vi "Lake Shore Cryotronics 218 Alarm Configuration.vi"() -> ()   [LabVIEW 2017]
doc: "This example VI demonstrates the use of the Alarm VIs to configure the Alarm function and monitor the Alarm Status for the selected input. A typical use of this example would be to configure the Alarm functions the first time this is run and then monitor the Alarm status by running this VI in a loop."
uses:
  Lake Shore Cryotronics 218.lvlib
panel:
  out "VISA resource name out":refnum<visa-resource-name>
  out "error out":errorcluster
  in  "error in (no error)":errorcluster
  in  "VISA resource name":refnum<visa-resource-name>
  out "Beeper Status (F)":bool
  out "Alarm Low Status (F)":bool
  out "Alarm High Status (F)":bool
  in  "Beeper (F: Beeper Disabled)":bool
  in  "Latching (F: Alarm Latch OFF)":bool
  in  "Alarm (F: Alarm Disabled)":bool
  in  "Deadband (0.0000)":dbl min=0.0 max=9999.9 step=0.0001 format="%.4f"
  in  "Low Value (0.0000)":dbl min=-9999.9 max=9999.9 step=0.0001 format="%.4f"
  in  "High Value (0.0000)":dbl min=-9999.9 max=9999.9 step=0.0001 format="%.4f"
  in  "Alarm Source (0:Kelvin)":u16(ring) items=["Kelvin", "Celsius", "Sensor Units", "Linear Data"]
  in  "Input (1)":dbl=1.0 min=1.0 max=8.0 step=1.0
  in  "Configure/Read (Config:F)":bool
  # "© 2005 National Instruments.  ALL RIGHTS RESERVED."
  # "Configure Alarm"
  # "Read Alarm Status"
  # "Alarm Configuration"
  # "Alarm Status"
  # "High Alarm Active\nHigh Alarm Inactive"
  # "Alarm Enabled\nAlarm Disabled"
  # "Alarm Latch ON\nAlarm Latch OFF"
  # "Low Alarm Active\nLow Alarm Inactive"
  # "Beeper Enabled\nBeeper Disabled"
  # "Beeper Active\nBeeper Inactive"
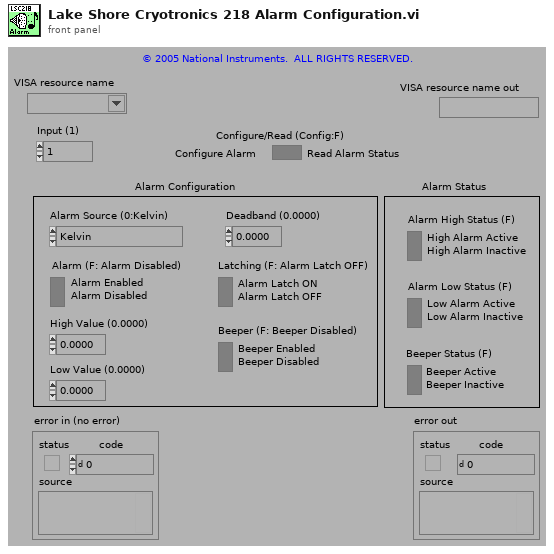
[diagram p1: front panel]
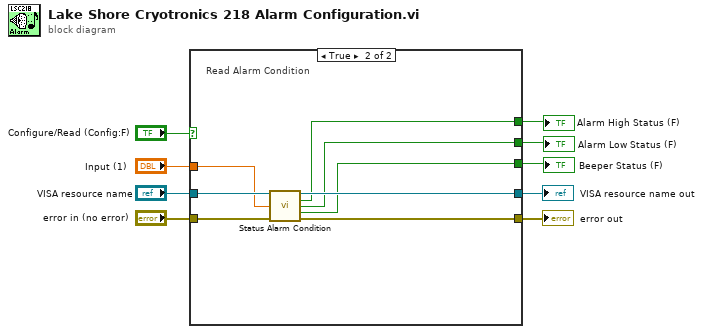
[diagram p0: block diagram]
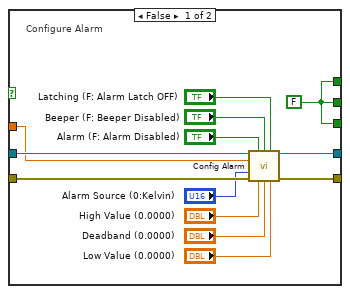
[diagram p2: hidden frame]
diagram:
  n1 = case shown="True" "Configure/Read (Config:F)" {
    tunnel: "error in (no error)" -> [w19 w29]
    tunnel: "VISA resource name" -> [w20 w30]
    tunnel: [w21 w27] -> w5
    tunnel: "Input (1)" -> [w18 w26]
    tunnel: [w22 w28] -> w4
    tunnel: [w10 w25] -> w3
    tunnel: [w10 w24] -> w2
    tunnel: [w10 w23] -> w1
    frame False {
      w10 = FALSE ("Alarm High/Low & Beeper Status")
      # "Configure Alarm"
      n2 = call "Config Alarm.vi"("VISA resource name"=w20, "Alarm (F: Alarm Disabled)"="Alarm (F: Alarm Disabled)", "Beeper (F: Beeper Disabled)"="Beeper (F: Beeper Disabled)", "Latching (F: Alarm Latch OFF)"="Latching (F: Alarm Latch OFF)", "Input (1)"=w18, "Alarm Source (0:Kelvin)"="Alarm Source (0:Kelvin)", "error in (no error)"=w19, "High Value (0.0000)"="High Value (0.0000)", "Deadband (0.0000)"="Deadband (0.0000)", "Low Value (0.0000)"="Low Value (0.0000)") -> ("VISA resource name out"=w21:refnum<visa-resource-name>, "error out"=w22:errorcluster)  [unwired: 4 in]
    }
    frame True {
      # "Read Alarm Condition"
      n3 = call "Status Alarm Condition.vi"("VISA resource name"=w30, "Input (1)"=w26, "error in (no error)"=w29) -> ("VISA resource name out"=w27:refnum<visa-resource-name>, "Alarm High Status"=w23:bool, "Alarm Low Status"=w24:bool, "Beeper Status"=w25:bool, "error out"=w28:errorcluster)  [unwired: 8 in]
    }
  }
  "VISA resource name out" <- w5
  "error out" <- w4
  "Beeper Status (F)" <- w3
  "Alarm Low Status (F)" <- w2
  "Alarm High Status (F)" <- w1
